vi "ChangeSampleFlow.vi"(7 "LVWS Req":refnum<class "Web Request.lvclass">, 11 "State":u8) -> ()   [LabVIEW 2014]
doc: "Service for changing the direction of the flow: 0 = cabn, 1 = inlet."
uses:
  <vilib>/wsapi/Web Request.lvclass
  Controller/Messages/Change Inlet MSG/Change Inlet MSG.lvclass
  Controller/Messages/Change Inlet MSG/Change Inlet MSG.lvclass/Change Inlet MSG.ctl
  Controller/Messages/Change Inlet MSG/Write Cabin.vi
  Controller/Controller.lvclass
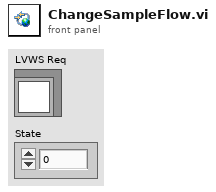
[diagram p1: front panel]
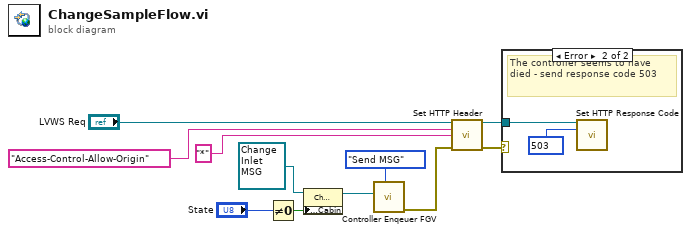
[diagram p0: block diagram]
diagram:
  n1 = Not Equal To 0?(x="State") -> (x != 0?=w5:bool)
  n2 = property class="Change Inlet MSG.lvclass"(reference=refnum<class "Change Inlet MSG.lvclass"> refnum ("Controller.lvlib:Change Inlet MSG.lvclass"), "Accessors:Cabin"=w5) -> (reference out=w4:refnum<class "Change Inlet MSG.lvclass">)  [unwired: 1 in, 1 out]
  n3 = call "Controller Enqeuer FGV.vi"("State"=enum16{"Store", "Send MSG"}."Send MSG", "MSG"=w4) -> ("error out"=w2:errorcluster)  [unwired: 9 in]
  n4 = call <vilib>:"Set HTTP Header.vi"("LabVIEW Web Service Request"="LVWS Req", "header"="Access-Control-Allow-Origin", "header value"="*", "error in (no error)"=w2) -> ("LabVIEW Web Service Request out"=w9:refnum<class "Web Request.lvclass">, "error out"=w1:errorcluster)  [unwired: 10 in]
  n5 = case shown="Error" w1 {
    tunnel: w9 -> [_ w12]
    frame No Error {
    }
    frame Error {
      w13 = 503 items=["100"=100, "101"=101, "200"=200, "201"=201, "202"=202, "203"=203, "204"=204, "205"=205, "206"=206, "300"=300, "301"=301, "302"=302, "303"=303, "304"=304, "305"=305, "306"=306, "307"=307, "400"=400, "401"=401, "402"=402, "403"=403, "404"=404, "405"=405, "406"=406, "407"=407, "408"=408, "409"=409, "410"=410, "411"=411, "412"=412, "413"=413, "414"=414, "415"=415, "416"=416, "417"=417, "500"=500, "501"=501, "502"=502, "503"=503, "504"=504, "505"=505] ("response code (200)")
      # "The controller seems to have died - send response code 503"
      n6 = call <vilib>:"Set HTTP Response Code.vi"("LabVIEW Web Service Request"=w12, "response code (200)"=w13) -> ()  [unwired: 12 in, 2 out]
    }
  }
